vi "enqueue readings.vi"(8 "error in":errorcluster, 9 "crrossing elements in":u32, 10 "readings from serial":T1[](array[typedef]), 11 "queues":T3[](array[typedef])) -> (0 "error out":errorcluster, 1 "crossing elements read":u32, 3 "last pulse":T1, 4 "mag set working out":bool[](array[boolean]))   [LabVIEW 2017]
uses:
  typedefs/reading.ctl
  typedefs/readingType.ctl
  typedefs/queue cluster.ctl
  typedefs/reading queue.ctl
  typedefs/magnetomter reading set.ctl
  typedefs/orbit parameters with crossing info.ctl
  typedefs/magnet location with timestamp.ctl
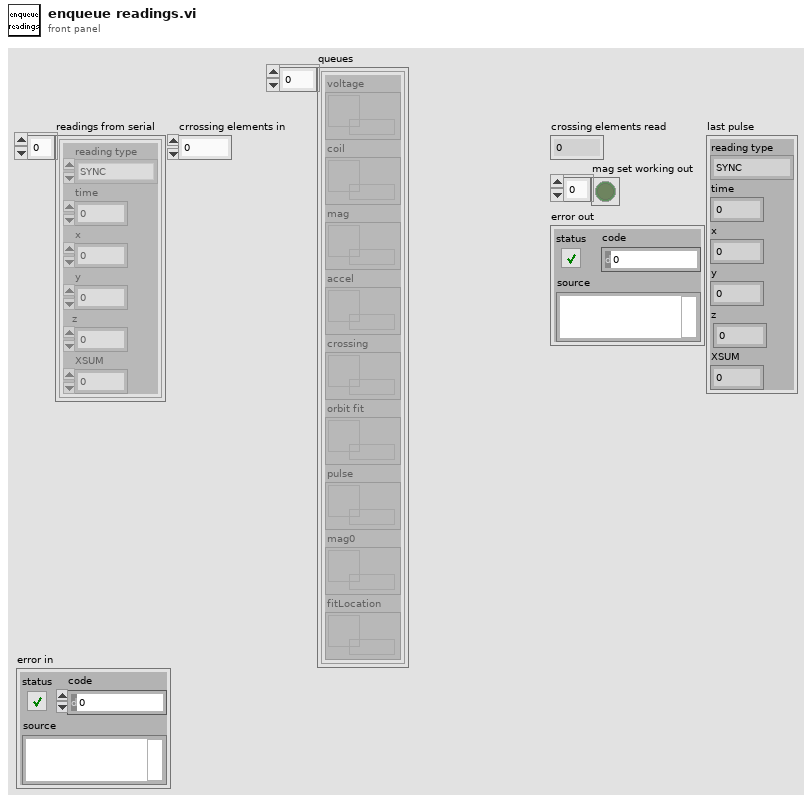
[diagram p1: front panel]
types:
  T1 = typedef "reading.ctl" = cluster{"reading type":T2, "time":fxp<+,48,48>, "x":sgl, "y":sgl, "z":sgl, "XSUM":u8}
  T2 = typedef "readingType.ctl" = enum8{"SYNC", "DETVAL", "COILI", "MAGVEC", "ACCVEC", "CROSSING", "MAGVEC0", "MAGVEC1", "MAGVEC2", "MAGVEC3", "MAGVEC4", "MAGVEC5", "MAGVEC6", "MAGVEC7"}
  T3 = typedef "queue cluster.ctl" = cluster{"voltage":T4, "coil":T4, "mag":refnum<queue>, "accel":T4, "crossing":T4, "orbit fit":refnum<queue>, "pulse":T4, "mag0":T4, "fitLocation":refnum<queue>}
  T4 = typedef "reading queue.ctl" = refnum<queue>
  T5 = typedef "magnetomter reading set.ctl" = cluster{"time":fxp<+,48,48>, "mag readings":cluster{"magnetometer index":dbl, "Bx":dbl, "By":dbl, "Bz":dbl, "magnetometer x":dbl, "magnetometer y":dbl}[]}
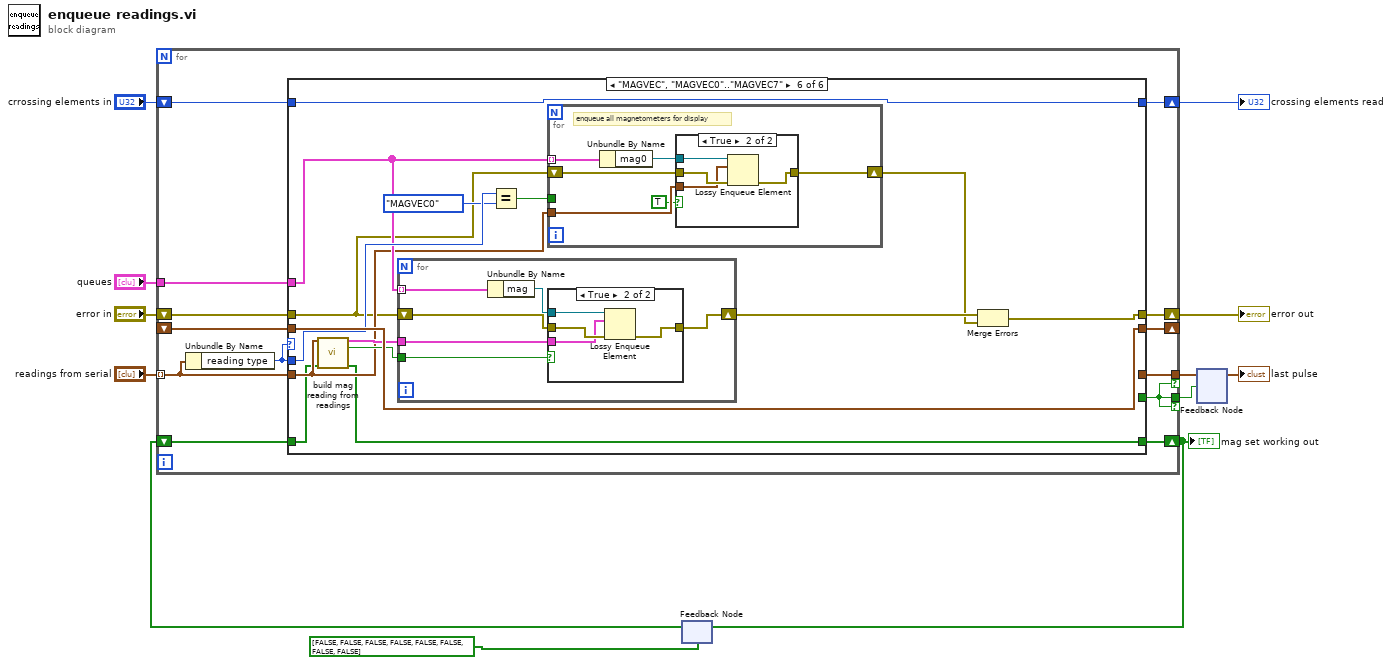
[diagram p0: block diagram]
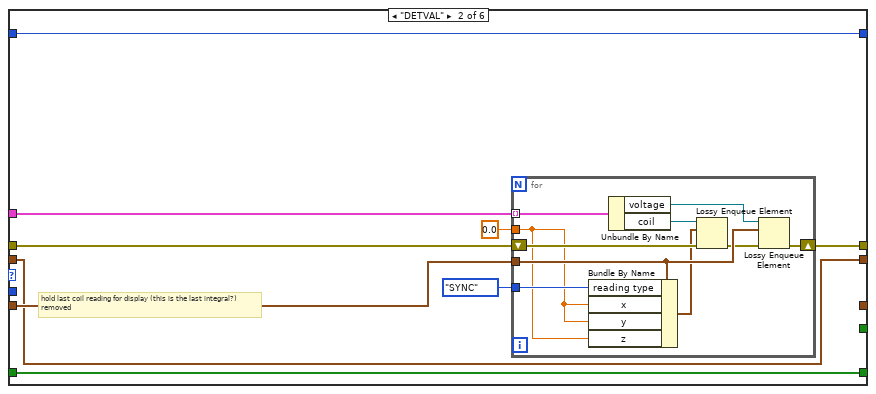
[diagram p3: hidden frame]
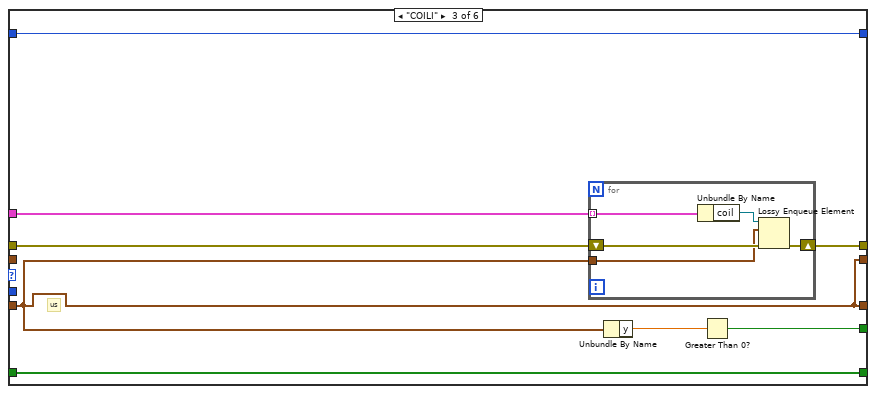
[diagram p4: hidden frame]
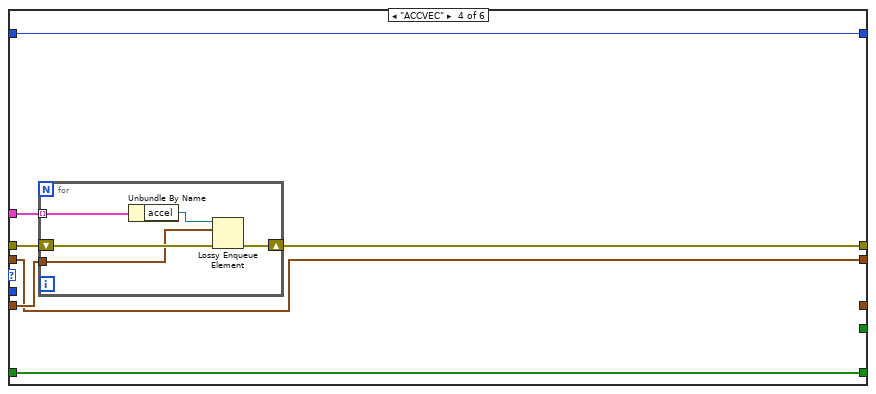
[diagram p5: hidden frame]
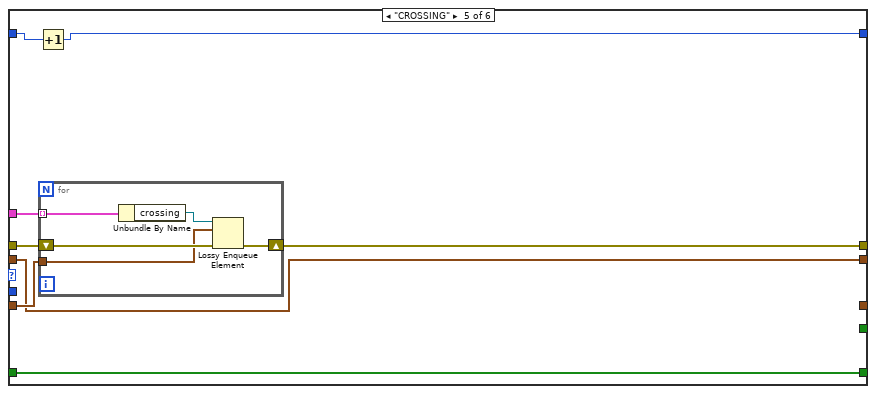
[diagram p6: hidden frame]
diagram:
  n1 = feedback #1(bool[] [FALSE, FALSE, FALSE, FALSE, FALSE, FALSE, FALSE, FALSE] ("mag set working out")) -> (w2:bool[])
  n2 = for {
    tunnel: "readings from serial" -> [w16] mode=indexing
    tunnel: "queues" -> [w24]
    shift-right: [w23] -> w9
    shift-left: "error in" -> [w25]
    shift-right: [w21] -> w7
    shift-left: "crrossing elements in" -> [w22]
    shift-right: [w20] -> _
    shift-left: _ -> [w19]
    tunnel: [w18] -> w6 if=w17
    tunnel: [w17] -> w4 if=w17
    shift-right: [w14] -> w3
    shift-left: w2 -> [w13]
    n3 = Unbundle By Name(w16) -> ("reading type"=w15:T2)
    n4 = case shown="\"MAGVEC\", \"MAGVEC0\"..\"MAGVEC7\"" w15 {
      tunnel: w16 -> [_ w34 w50 w65 w78 w93]
      tunnel: w25 -> [w29 w32 w56 w68 w81 w91]
      tunnel: w24 -> [_ w38 w55 w67 w80 w94]
      tunnel: [w29 w37 w54 w66 w79 w90] -> w23
      tunnel: w22 -> [w28 w36 w53 w64 w77 w100]
      tunnel: [w28 w36 w53 w64 w76 w100] -> w21
      tunnel: [w27 w33 w50 w63 w75 w99] -> w20
      tunnel: w19 -> [w27 w33 _ w63 w75 w99]
      tunnel: [_ _ w51 _ _ _] -> w17
      tunnel: [_ _ w50 _ _ _] -> w18
      tunnel: w15 -> [_ _ _ _ _ w96]
      tunnel: [w26 w30 w49 w62 w74 w88] -> w14
      tunnel: w13 -> [w26 w30 w49 w62 w74 w87]
      frame "SYNC", Default {
      }
      frame "DETVAL" {
        # "hold last coil reading for display (this is the last integral?)\nremoved"
        n5 = for {
          tunnel: w38 -> [w47] mode=indexing
          tunnel: readingType."SYNC" ("reading type") -> [w45]
          tunnel: w34 -> [w44]
          tunnel: sgl 0.0 ("x") -> [w40]
          shift-right: [w46] -> w37
          shift-left: w32 -> [w43]
          n6 = Bundle By Name(cluster=w44, "reading type"=w45, "x"=w40, "y"=w40, "z"=w40) -> (w39:T1)
          n7 = Unbundle By Name(w47) -> ("voltage"=w48:T4, "coil"=w41:T4)
          n8 = Lossy Enqueue Element(queue=w41, element=w39, error in (no error)=w43) -> (error out=w42:errorcluster)  [unwired: 3 out]
          n9 = Lossy Enqueue Element(queue=w48, element=w44, error in (no error)=w42) -> (error out=w46:errorcluster)  [unwired: 3 out]
        }
      }
      frame "COILI" {
        # "us"
        n10 = for {
          tunnel: w55 -> [w60] mode=indexing
          tunnel: w50 -> [w57]
          shift-right: [w59] -> w54
          shift-left: w56 -> [w61]
          n11 = Unbundle By Name(w60) -> ("coil"=w58:T4)
          n12 = Lossy Enqueue Element(queue=w58, element=w57, error in (no error)=w61) -> (error out=w59:errorcluster)  [unwired: 3 out]
        }
        n13 = Unbundle By Name(w50) -> ("y"=w52:sgl)
        n14 = Greater Than 0?(x=w52) -> (x > 0?=w51:bool)
      }
      frame "ACCVEC" {
        n15 = for {
          tunnel: w67 -> [w71] mode=indexing
          tunnel: w65 -> [w69]
          shift-right: [w70] -> w66
          shift-left: w68 -> [w72]
          n16 = Unbundle By Name(w71) -> ("accel"=w73:T4)
          n17 = Lossy Enqueue Element(queue=w73, element=w69, error in (no error)=w72) -> (error out=w70:errorcluster)  [unwired: 3 out]
        }
      }
      frame "CROSSING" {
        n18 = Increment(x=w77) -> (x+1=w76:u32)
        n19 = for {
          tunnel: w80 -> [w84] mode=indexing
          tunnel: w78 -> [w82]
          shift-right: [w83] -> w79
          shift-left: w81 -> [w85]
          n20 = Unbundle By Name(w84) -> ("crossing"=w86:T4)
          n21 = Lossy Enqueue Element(queue=w86, element=w82, error in (no error)=w85) -> (error out=w83:errorcluster)  [unwired: 3 out]
        }
      }
      frame "MAGVEC", "MAGVEC0".."MAGVEC7" {
        n22 = call "build mag reading from readings.vi"("reading"=w93, "magnetometer set working in"=w87) -> ("reading out"=w98:T5, "reading completed"=w97:bool, "mag set working out"=w88:bool[])  [unwired: 11 in]
        n23 = for {
          tunnel: w94 -> [w117] mode=indexing
          tunnel: w98 -> [w114]
          tunnel: w97 -> [w113]
          shift-right: [w115] -> w101
          shift-left: w91 -> [w116]
          n24 = Unbundle By Name(w117) -> ("mag"=w118:refnum<queue>)
          n25 = case shown="True" w113 {
            tunnel: w118 -> [_ w123]
            tunnel: w116 -> [w119 w122]
            tunnel: [w119 w121] -> w115
            tunnel: w114 -> [_ w120]
            frame False {
            }
            frame True {
              n26 = Lossy Enqueue Element(queue=w123, element=w120, error in (no error)=w122) -> (error out=w121:errorcluster)  [unwired: 3 out]
            }
          }
        }
        n27 = Equal?(x=w96, y=readingType."MAGVEC0") -> (x = y?=w92:bool)
        n28 = for {
          tunnel: w93 -> [w104]
          tunnel: w92 -> [_]
          shift-right: [w105] -> w89
          shift-left: w91 -> [w106]
          tunnel: w94 -> [w103] mode=indexing
          # "enqueue all magnetometers for display"
          n29 = Unbundle By Name(w103) -> ("mag0"=w107:T4)
          n30 = case shown="True" TRUE {
            tunnel: w107 -> [_ w112]
            tunnel: w106 -> [w108 w111]
            tunnel: [w108 w110] -> w105
            tunnel: w104 -> [_ w109]
            frame False {
            }
            frame True {
              n31 = Lossy Enqueue Element(queue=w112, element=w109, error in (no error)=w111) -> (error out=w110:errorcluster)  [unwired: 3 out]
            }
          }
        }
        n32 = Merge Errors(w101, w89) -> (w90:errorcluster)
      }
    }
  }
  "error out" <- w9
  "crossing elements read" <- w7
  "mag set working out" <- w3
  n33 = feedback-in #1(w3) -> ()
  n34 = feedback-in #2(w6, w4) -> ()
  n35 = feedback #2() -> (→"last pulse":T1)  [unwired: 1 in]
